vi "ED_GetResponse.vi"(4 "error in (no error)":errorcluster, 7 "connection ID":refnum<k5>) -> (0 "error out":errorcluster, 2 "response":string, 3 "connection ID out":refnum<k5>)   [LabVIEW 2013, in "CAENels EASY-DRIVER.lvlib"]
uses:
  <instrlib>/CAENels EASY-DRIVER/CAENels EASY-DRIVER.lvlib
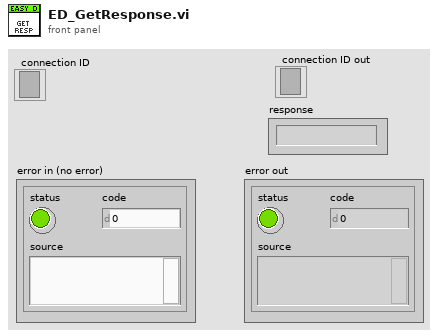
[diagram p1: front panel]
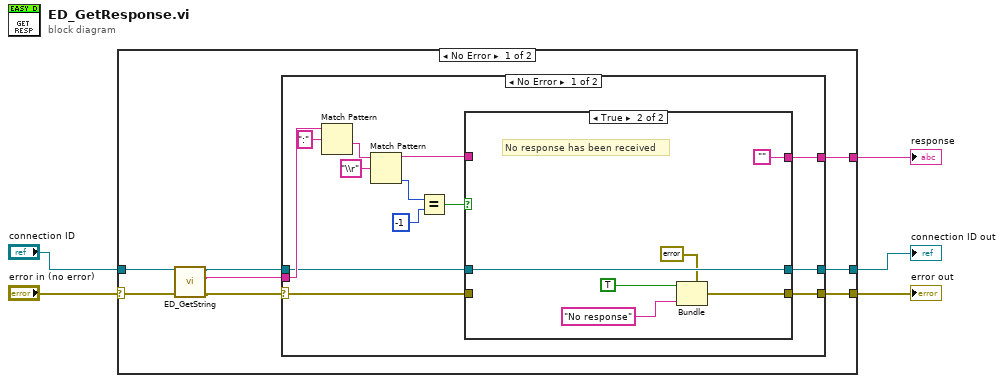
[diagram p0: block diagram]
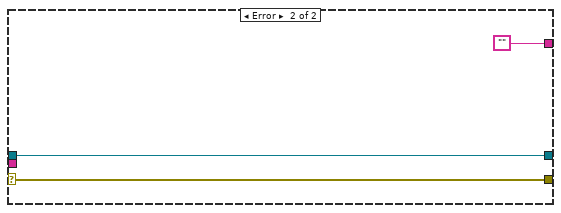
[diagram p3: hidden frame]
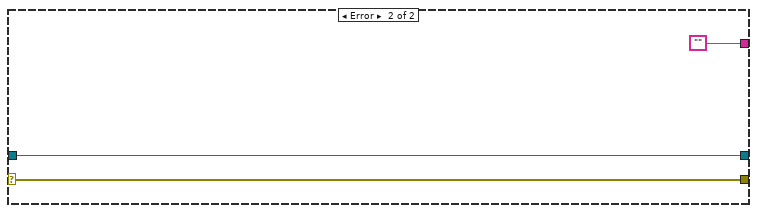
[diagram p4: hidden frame]
diagram:
  n1 = case shown="No Error" "error in (no error)" {
    selector: "error in (no error)" -> [w9 w41]
    tunnel: "connection ID" -> [w10 w40]
    tunnel: [w13 w41] -> w3
    tunnel: [w12 w40] -> w2
    tunnel: [w11 ""] -> w1
    frame No Error {
      n2 = call <instrlib>:"ED_GetString.vi"("error in"=w9, "connection ID in"=w10) -> ("error out"=w7:errorcluster, "String"=w6:string, "connection ID out"=w8:refnum<k5>)  [unwired: 3 in]
      n3 = case shown="No Error" w7 {
        selector: w7 -> [w23 w38]
        tunnel: [w22 w38] -> w13
        tunnel: [w20 w37] -> w12
        tunnel: w8 -> [w21 w37]
        tunnel: w6 -> [w26 _]
        tunnel: [w14 ""] -> w11
        frame No Error {
          n4 = Match Pattern(string=w26, regular expression=":") -> (after substring=w18:string)  [unwired: 4 out]
          n5 = Match Pattern(string=w18, regular expression="\\r") -> (before substring=w15:string, offset past match=w16:i32)  [unwired: 3 out]
          n6 = Equal?(x=w16, y=-1) -> (x = y?=w24:bool)
          n7 = case shown="True" w24 {
            tunnel: [w29 w34] -> w22
            tunnel: w23 -> [w29 _]
            tunnel: w21 -> [w28 w35]
            tunnel: [w28 w35] -> w20
            tunnel: [w27 ""] -> w14
            tunnel: w15 -> [w27 _]
            frame False {
              # "Response has been found"
            }
            frame True {
              # "No response has been received"
              n8 = Bundle(cluster=errorcluster {"status"=FALSE, "code"=0, "source"=""} ("error in  2"), "status"=TRUE, "source"="No response") -> (w34:errorcluster)  [unwired: 1 in]
            }
          }
        }
        frame Error {
        }
      }
    }
    frame Error {
    }
  }
  "error out" <- w3
  "connection ID out" <- w2
  "response" <- w1
